vi "State_Machine.vi"(8 "error in (no error)":errorcluster caption="entrée d'erreur (pas d'erreur)", 11 "Get_Voltage en entrée":refnum<class "Zigbee_Send_Msg_Manufacturer_Name.lvclass">) -> (0 "error out":errorcluster caption="sortie d'erreur", 2 "Json_String":string, 3 "Get_Voltage en sortie":refnum<class "Zigbee_Send_Msg_Manufacturer_Name.lvclass">)   [LabVIEW 2020, in "Library Test.lvlib" / "Zigbee_Send_Msg_Manufacturer_Name.lvclass"]
uses:
  Zigbee_Send_Msg_Manufacturer_Name.lvclass
  C:/Users/rbruneau/Documents/Standard TB/Class/Test/Zigbee_Send_Msg/Zigbee_Send_Msg.lvclass
  Zigbee_Send_Msg/Zigbee_Send_Msg.lvclass
  Zigbee_Send_Msg_Manufacturer_Name.lvclass/Zigbee_Send_Msg_Manufacturer_Name.ctl
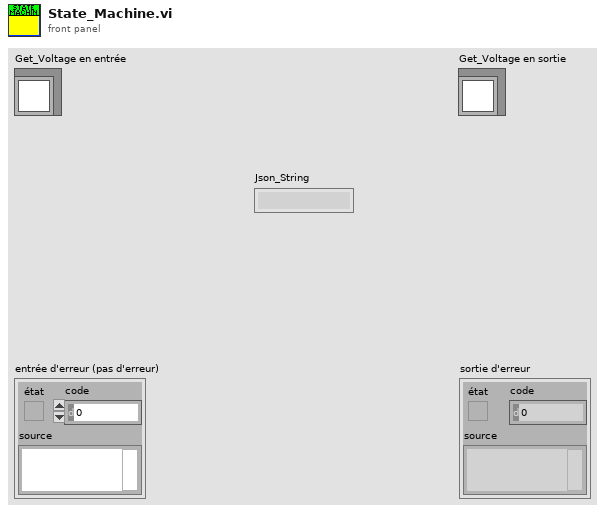
[diagram p1: front panel]
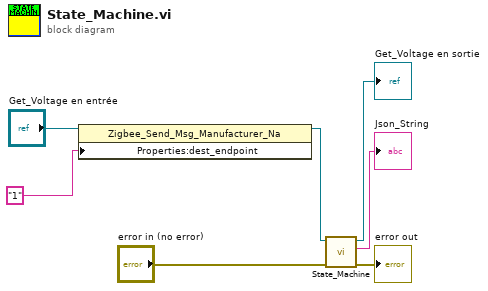
[diagram p0: block diagram]
diagram:
  n1 = property class="Zigbee_Send_Msg_Manufacturer_Na"(reference="Get_Voltage en entrée", "Properties:dest_endpoint"="1") -> (reference out=w2:refnum<class "Zigbee_Send_Msg_Manufacturer_Name.lvclass">)  [unwired: 1 in, 1 out]
  n2 = call-parent "State_Machine.vi"("error in (no error)"="error in (no error)", "Get_Voltage en entrée"=w2) -> ("error out"=→"error out":errorcluster, "Json_String"=→"Json_String":string, "Get_Voltage en sortie"=→"Get_Voltage en sortie":refnum<class "Zigbee_Send_Msg_Manufacturer_Name.lvclass">)  [unwired: 7 in]
